vi "Default Config--constant.vi"() -> (3 "Default Config":T1)   [LabVIEW 2020, in "MacroAssert.lvlib"]
uses:
  MacroAssert.lvlib
  CTLs/Config.ctl
  <vilib>/Utility/sysdir.llb/System Directory Type.ctl
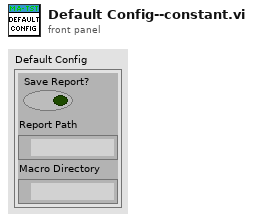
[diagram p1: front panel]
types:
  T1 = typedef "MacroAssert.lvlib/Config.ctl" = cluster{"Save Report?":bool, "Report Path":path, "Macro Directory":path}
  T2 = typedef "System Directory Type.ctl" = i32
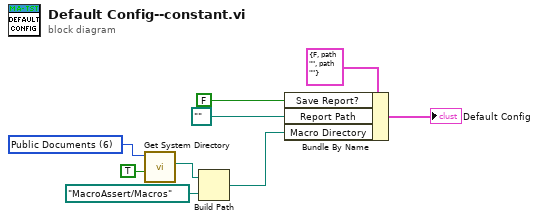
[diagram p0: block diagram]
diagram:
  w3 = T2 6 items=["User Home"=0, "User Desktop"=1, "User Documents"=2, "User Application Data"=3, "User Preferences"=4, "User Temporary"=5, "Public Documents"=6, "Public Application Data"=7, "Public Preferences"=8, "Public Cache"=13, "System Core Libraries"=9, "System Installed Libraries"=10, "Application Files"=11, "Boot Volume Root"=12] ("system directory type")
  n1 = call <vilib>:"Get System Directory.vi"("create directory if not found? (F)"=TRUE, "system directory type"=w3) -> ("system directory"=w5:path)  [unwired: 9 in]
  n2 = Build Path(base path=w5, name or relative path=path "MacroAssert/Macros") -> (appended path=w2:path)
  n3 = Bundle By Name(cluster=T1 {"Save Report?"=FALSE, "Report Path"=path "", "Macro Directory"=path ""} ("Config"), "Save Report?"=FALSE, "Report Path"=path "", "Macro Directory"=w2) -> (→"Default Config":T1)
